vi "PH_Countdown-Counter.PC PPInternalTiming.vi"(0 "i ref in":refnum<vi>, 2 "Servicename":string, 3 "Waiting Time [s]":i32=30, 4 "no link?":bool, 5 "error in (no error)":errorcluster) -> (14 "i ref out":refnum<vi>, 19 "error out":errorcluster)   [LabVIEW 2014, in "PH_Countdown-Counter.lvlib"]
doc: "This VI writes the remaining waiting time of the PU to own attributes and the GUI elements."
uses:
  PH_Countdown-Counter.lvlib
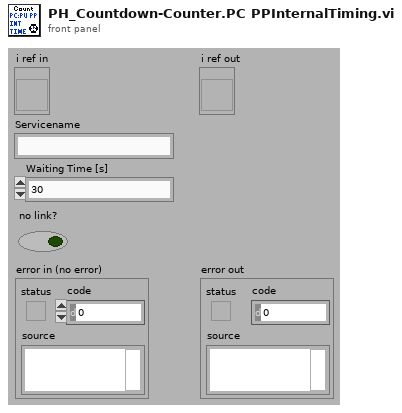
[diagram p1: front panel]
types:
  T1 = typedef "PH_Countdown-Counter.lvlib/PH_Countdown-Counter.i attribute.ctl" = cluster{"Machine Time":cluster{"Tag":string, "Wating Time [s]":dbl, "not linked?":bool}[], "Last Shot":cluster{"Tag":string, "Shot Time [s]":timestamp, "not linked?":bool}[], "Time since last Shot?":bool, "Calculation":cluster{"Time between Shots [s]":dbl, "Ref Remaining Time":refnum<vi>, "Service ID":i32, "over?":bool, "Ref Time between Shots":refnum<vi>, "Ref Set Mode":refnum<vi>}, "Sound?":bool, "Reminder":cluster{"# 1":cluster{"Pretime [s]":dbl, "Aktive?":bool, "Over?":bool}, "# 2":cluster{"Pretime [s]":dbl, "Aktive?":bool, "Over?":bool}}, "MainAmp only":cluster{"State":bool, "GUI Ref":refnum<vi>}}
  T2 = cluster{"Tag":string, "Wating Time [s]":dbl, "not linked?":bool}[]
  T3 = cluster{"Tag":string, "Wating Time [s]":dbl, "not linked?":bool}
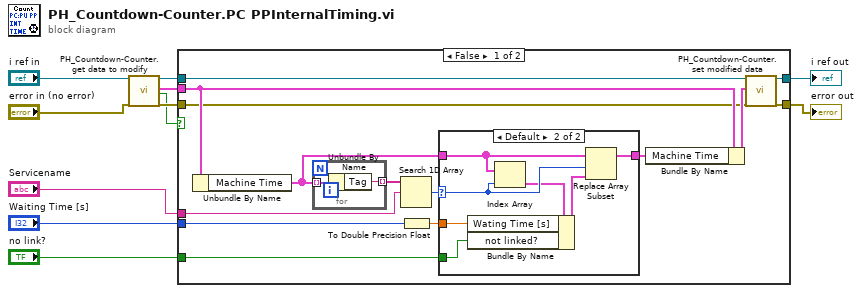
[diagram p0: block diagram]
diagram:
  n1 = call "PH_Countdown-Counter.get data to modify.vi"("i ref in"="i ref in", "error in (no error)"="error in (no error)") -> ("i ref out"=w7:refnum<vi>, "i attribute"=w4:T1, "timed out"=w1:bool, "error out"=w10:errorcluster)  [unwired: 14 in]
  n2 = case shown="False" w1 {
    tunnel: "Waiting Time [s]" -> [w25 _]
    tunnel: w10 -> [w12 w36]
    tunnel: w7 -> [w24 w37]
    tunnel: "Servicename" -> [w22 _]
    tunnel: "no link?" -> [w19 _]
    tunnel: w4 -> [w17 _]
    tunnel: [w15 w37] -> w3
    tunnel: [w13 w36] -> w2
    frame False {
      n3 = Unbundle By Name(w17) -> ("Machine Time"=w18:T2)
      n4 = for {
        tunnel: w18 -> [w35] mode=indexing
        tunnel: [w34] -> w23 mode=indexing
        n5 = Unbundle By Name(w35) -> ("Tag"=w34:string)
      }
      n6 = Search 1D Array(1D array=w23, element=w22) -> (index of element=w21:i32)  [unwired: 1 in]
      n7 = To Double Precision Float(number=w25) -> (double precision float=w20:dbl)
      n8 = case shown="Default" w21 {
        selector: w21 -> [_ w28]
        tunnel: w20 -> [_ w33]
        tunnel: w19 -> [_ w30]
        tunnel: w18 -> [w26 w29]
        tunnel: [w26 w31] -> w16
        frame -1 {
        }
        frame Default {
          n9 = Index Array(array=w29, index=w28) -> (element=w27:T3)
          n10 = Bundle By Name(cluster=w27, "Wating Time [s]"=w33, "not linked?"=w30) -> (w32:T3)
          n11 = Replace Array Subset(array=w29, new element=w32, index=w28) -> (w31:T2)
        }
      }
      n12 = Bundle By Name(cluster=w17, "Machine Time"=w16) -> (w14:T1)
      n13 = call "PH_Countdown-Counter.set modified data.vi"("i ref in"=w24, "i attribute"=w14, "error in (no error)"=w12) -> ("i ref out"=w15:refnum<vi>, "error out"=w13:errorcluster)  [unwired: 15 in]
    }
    frame True {
    }
  }
  "error out" <- w2
  "i ref out" <- w3
